vi "Initialize Log File.vi"(8 "error in (no error)":errorcluster, 11 "Path":path) -> (0 "error out":errorcluster)   [LabVIEW 2024]
uses:
  <vilib>/Utility/file.llb/Write Delimited Spreadsheet (string).vi
panel:
  in  "Headers":string[](array[string])=["timestamp", "event_name", "scenario", "counts_file#", "scattering_file#", "output_file#", "AI2_file#", "dio0", "dio1", "dio2", "dio3", "ch2", "ch2_mod", "ch2_ac_freq", "ch2_ac_volt", "ch2_mod_type", "ch2_mod_waveform", "ch2_mod_freq", "ch2_mod_depth", "threshold_value", "precheck_duration", "scenario_duration", "release_duration", "f_start", "f_end", "fc_start", "fc_end", "number_of_steps", "total_time", "depth_start", "depth_end", "modulation_ch", "amp_start", "amp_end", "DC offset"]
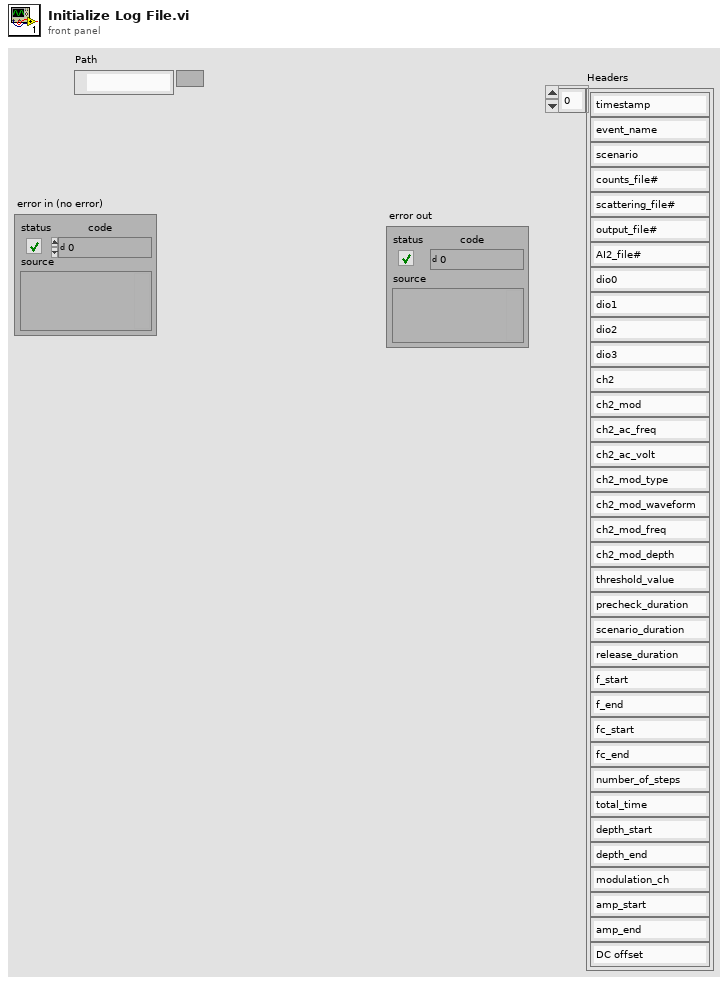
[diagram p1: front panel]
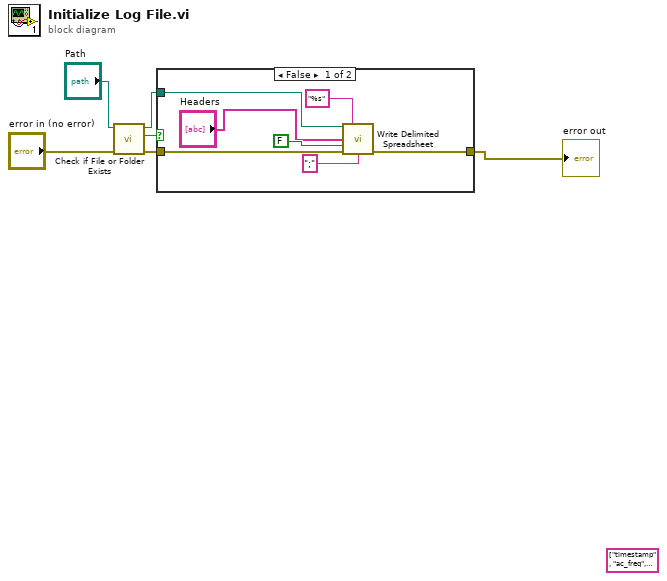
[diagram p0: block diagram]
diagram:
  (unwired) string[] ["timestamp", "ac_freq", "ac_volt", "mod_waveform", "mod_freq", "mod_depth", "dio0", "dio1", "dio2", "dio3"] ("Headers")
  n1 = call <vilib>:"Check if File or Folder Exists.vi"("error in (no error)"="error in (no error)", "path"="Path") -> ("error out"=w4:errorcluster, "file or folder exists?"=w5:bool, "dup path"=w1:path)  [unwired: 7 in]
  n2 = case shown="False" w5 {
    tunnel: w4 -> [w13 w14]
    tunnel: [w12 w14] -> w3
    tunnel: w1 -> [w8 _]
    frame False {
      n3 = call-poly <vilib>:"Write Delimited Spreadsheet.vi"("file path (dialog if empty)"=w8, "format (%s)"="%s" ("format (%.3f)"), "1D data"="Headers", "append to file? (new file:F)"=FALSE, "error in (no error)"=w13, "delimiter (\\t)"=";" ("delimiter (\\t)")) -> ("error out"=w12:errorcluster)  [unwired: 8 in, 1 out]
    }
    frame True {
    }
  }
  "error out" <- w3
